vi "QR Code Scan Dialog.vi"(8 "error in (no error)":errorcluster, 10 "Camera Settings":T2={"fps"=30, "compression"=30, "Image Size"=enum."640x480"}, 11 "Camera Address":string="USB 0") -> (0 "error out":errorcluster, 3 "Output":string)   [LabVIEW 2015]
uses:
  <vilib>/Rock Robotics/WPI/Camera/WPI_CameraSettings Read MJPG.ctl
  <vilib>/Rock Robotics/WPI/Camera/WPI_CameraImageSize.ctl
  <vilib>/Utility/error.llb/DialogType.ctl
panel:
  in  "Done":bool
  in  "Cancel Button":bool
  out "Image":T1(plugin-control)
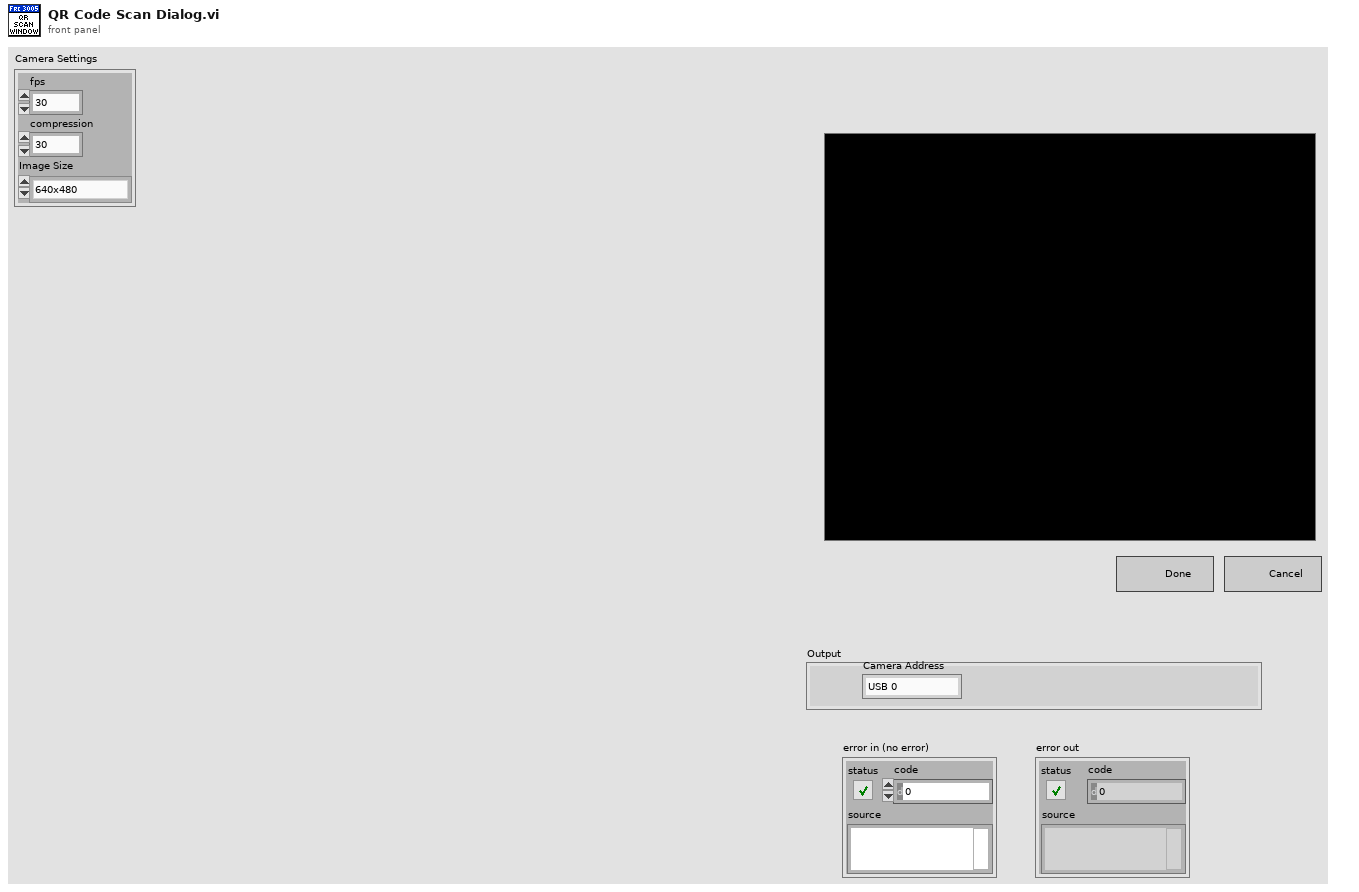
[diagram p1: front panel]
types:
  T1 = typedef "IMAQ Image.ctl" = refnum<image>
  T2 = typedef "WPI_CameraSettings Read MJPG.ctl" = cluster{"fps":i32, "compression":i32, "Image Size":T3}
  T3 = typedef "WPI_CameraImageSize.ctl" = enum16{"640x480", "320x240", "160x120", "Custom"}
  T4 = typedef "DialogType.ctl" = u16
  T5 = typedef "Image Type" = u32
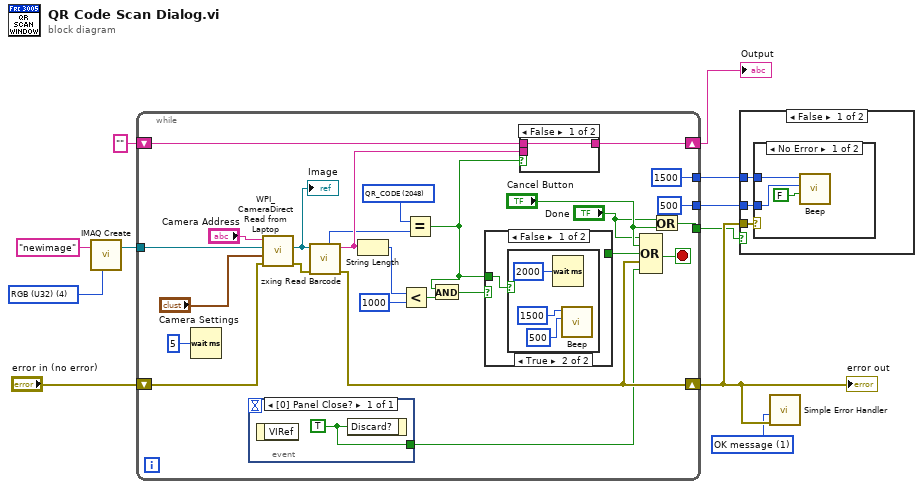
[diagram p0: block diagram]
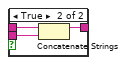
[diagram p4: hidden frame]
diagram:
  w4 = T4 1 items=["no dialog", "OK message", "continue or stop message", "OK message + warnings", "continue/stop + warnings"] ("type of dialog (OK msg:1)")
  w9 = T5 4 items=["Grayscale (U8)", "Grayscale (I16)", "Grayscale (SGL)", "Complex (CSG)", "RGB (U32)", "HSL (U32)", "RGB (U64)", "Grayscale (U16)"] ("Image Type")
  n1 = call "IMAQ Create"("Image Name"="newimage", "Image Type"=w9) -> ("New Image"=w10:T1)  [unwired: 3 in, 1 out]
  n2 = while {
    tunnel: w10 -> [w34]
    tunnel: [u32 1500 ("frequency (Hz)")] -> w8
    tunnel: [u32 500 ("frequency (Hz)")] -> w7
    shift-right: [w27] -> w5
    shift-left: "error in (no error)" -> [w29]
    tunnel: [w14] -> w3
    shift-right: [w18] -> w1
    shift-left: "" -> [w19]
    stop <- w30 stop-if-true
    w15 = 2048 items=["AZTEC"=1, "CODABAR"=2, "CODE_39"=4, "CODE_93"=8, "CODE_128"=16, "DATA_MATRIX"=32, "EAN_8"=64, "EAN_13"=128, "ITF"=256, "MAXICODE"=512, "PDF_417"=1024, "QR_CODE"=2048, "RSS_14"=4096, "RSS_EXPANDED"=8192, "UPC_A"=16384, "UPC_E"=32768, "UPC_EAN_EXTENSION"=65536, "MSI"=131072, "All_1D"=192990, "PLESSEY"=262144] ("BarcodeFormat")
    n3 = Wait (ms)(milliseconds to wait=u32 5) -> ()  [unwired: 1 out]
    n4 = event shown="[0] Panel Close?" {
      selector: _ -> [_]
      dyn-events: _ -> [_]
      timeout: _ -> [_]
      tunnel: [w38] -> w12
      event Panel Close? {
        w38 = TRUE ("Discard?")
        n5 = event-data() -> ()  [unwired: 1 in, 1 out]
        n6 = event-data("Discard?"=w38) -> ()  [unwired: 1 in, 1 out]
      }
    }
    n7 = call <vilib>:"WPI_CameraDirect Read from Laptop.vi"("error in"=w29, "Camera Settings"="Camera Settings", "Image"=w34, "address"="Camera Address") -> ("error out"=w28:errorcluster, "Image Out"=w31:T1)  [unwired: 6 in]
    "Image" <- w31
    n8 = call "zxing Read Barcode.vi"("error in (no error)"=w28, "Image"=w31) -> ("error out"=w27:errorcluster, "Text"=w20:string, "BarcodeFormat"=w16:i32)  [unwired: 7 in]
    n9 = String Length(string=w20) -> (length=w24:i32)
    n10 = Less?(x=w24, y=1000) -> (x < y?=w23:bool)
    n11 = Equal?(x=w15, y=w16) -> (x = y?=w17:bool)
    n12 = And(x=w17, y=w23) -> (x .and. y?=w25:bool)
    n13 = case shown="False" w25 {
      tunnel: w17 -> [w43 w47]
      tunnel: [_ w47] -> w21
      frame False {
        n14 = case shown="True" w43 {
          frame False {
          }
          frame True {
            n15 = Wait (ms)(milliseconds to wait=u32 2000) -> ()  [unwired: 1 out]
            n16 = call <vilib>:"Beep.vi"("duration (msec)"=u32 500 ("frequency (Hz)"), "frequency (Hz)"=u32 1500) -> ()  [unwired: 10 in]
          }
        }
      }
      frame True {
      }
    }
    n17 = case shown="False" w17 {
      tunnel: w20 -> [_ w42]
      tunnel: w19 -> [w39 w41]
      tunnel: [w39 w40] -> w18
      frame False {
      }
      frame True {
        n18 = Concatenate Strings(w41, w42) -> (w40:string)
      }
    }
    n19 = Compound Arithmetic op=OR("Done", "Cancel Button", w21, w27, w12) -> (w30:bool)
    n20 = Or(x="Done", y="Cancel Button") -> (x .or. y?=w14:bool)
  }
  "error out" <- w5
  "Output" <- w1
  n21 = case shown="False" w3 {
    tunnel: w8 -> [w50 _]
    tunnel: w7 -> [w49 _]
    tunnel: w5 -> [w48 _]
    frame False {
      n22 = case shown="No Error" w48 {
        tunnel: w50 -> [w53 _]
        tunnel: w49 -> [w52 _]
        frame No Error {
          n23 = call <vilib>:"Beep.vi"("use system alert? (T)"=FALSE, "duration (msec)"=w52, "frequency (Hz)"=w53) -> ()  [unwired: 9 in]
        }
        frame Error {
        }
      }
    }
    frame True {
    }
  }
  n24 = call <vilib>:"Simple Error Handler.vi"("type of dialog (OK msg:1)"=w4, "error in (no error)"=w5) -> ()  [unwired: 3 in, 5 out]
